vi "CTL_TestController.vi"(6 "error in (no error)":errorcluster, 7 "VISA Refnum In":refnum<visa-resource-name>, 8 "TEST State In":T6, 11 "FullConfig":T7={"Bench Params"={"Relative Root Name"="PWC-OLS", "Values"={"Step Levels"=11.0, "Resistor Tolerence"=0.01, "Sample Rate"=0.05, "Resistor"=100.0, "Wait Time"=3.0}, "Report Template path"=path "PWC-OLS/$ReportFiles/ReportTemplate_03.xlsx", "Test Type"="OLS001", "Config File Name"="8005571-05 Elevate OLS .csv", "Config 2 Use"="Default", "Skip Pre Lube"=FALSE}, "Test Params"=[[98.0, 102.0, 8.5, 8.5, 8.5, 8.5, 98.0, 102.0, 8.5, 8.5, 8.5, 8.5], [98.0, 102.0, 7.91, 8.01, 7.55, 7.65, 98.0, 102.0, 7.685, 7.785, 7.325, 7.425], [197.0, 203.0, 7.46, 7.56, 7.1, 7.2, 197.0, 203.0, 7.235, 7.335, 6.875, 6.975], [296.0, 304.0, 7.01, 7.11, 6.65, 6.75, 296.0, 304.0, 6.785, 6.885, 6.425, 6.525], [395.0, 405.0, 6.56, 6.66, 6.2, 6.3, 395.0, 405.0, 6.335, 6.435, 5.975, 6.075], [494.0, 506.0, 6.11, 6.21, 5.75, 5.85, 494.0, 506.0, 5.885, 5.985, 5.525, 5.625], [593.0, 607.0, 5.66, 5.76, 5.3, 5.4, 593.0, 607.0, 5.435, 5.535, 5.075, 5.175], [692.0, 708.0, 5.21, 5.31, 4.85, 4.95, 692.0, 708.0, 4.985, 5.085, 4.625, 4.725], [791.0, 809.0, 4.76, 4.86, 4.4, 4.5, 791.0, 809.0, 4.535, 4.635, 4.175, 4.275], [890.0, 910.0, 4.31, 4.41, 3.95, 4.05, 890.0, 910.0, 4.085, 4.185, 3.725, 3.825], [989.0, 1011.0, 3.86, 3.96, 3.5, 3.6, 989.0, 1011.0, 3.635, 3.735, 3.275, 3.375], [1088.0, 1112.0, 3.41, 3.51, 3.05, 3.15, 1088.0, 1112.0, 3.185, 3.285, 2.825, 2.925], [1088.0, 1112.0, 2.5, 2.5, 2.5, 2.5, 1088.0, 1112.0, 2.5, 2.5, 2.5, 2.5]], "Pump Params"={"Empty Inches"=8.4, "Full Inches"=2.6, "RNG_SLOW"=0.5, "RNG_CREEP"=0.007, "RNG_STOP "=0.002, "VISA resource name"="Default", "SPD_SLOW"=1, "SPD_CREEP"=0, "SPD_FAST"=5, "Zero template"=path "30", "zero  Settle sec"=100, "Laser Slope"=-0.996, "Laser Offset"=9.601, "Sim Fill Rate"=0.002, "Cal Date"="CAL_Level_RnR_241105.xlsx", "Cal Technician"="7"}, "DataQ Params"={"Visa Name"="COM4", "Num Chan"=2, "Cal Coef"=[{"M"=175.33, "B"=2.65678}, {"M"=174.448, "B"=3.00272}, {"M"=175.0, "B"=3.0}, {"M"=175.0, "B"=3.0}, {"M"=175.0, "B"=3.0}, {"M"=175.0, "B"=3.0}, {"M"=175.0, "B"=3.0}, {"M"=175.0, "B"=3.0}], "Scale "=2, "Cal Date"="1/26/2024", "Cal Technicain"="Default"}, "Pump Control Ref"={"Fill "=refnum, "Drain"=refnum, "Level PV"=refnum, "Pump Speed"=refnum, "Run Test"=refnum, "Sim"=refnum, "Jog"=refnum, "Level SP"=refnum}, "Bench Status"={"Pump Status"=refnum, "Dataq Status"=refnum, "LaserStatus"=refnum}} {"Pump Params"."Sim Fill Rate" format="%.3f"; "Pump Params"."Laser Offset" format="%.3f"; "Pump Params"."Laser Slope" format="%.3f"; "Pump Params"."RNG_STOP" format="%#_13g"; "Pump Params"."RNG_CREEP" format="%#_13g"; "Pump Params"."RNG_SLOW" format="%#_13g"}) -> (0 "TEST State Out":T6, 1 "Enable":bool, 2 "Level Out":T1={"Laser "={"Raw"=0.0, "Scaled"=0.0}, "Level PV"=9.399999618530273, "Fill"=FALSE, "Drain"=FALSE}, 3 "Specs Out":T2={"aSpecsTable"=[], "Pump CtlRef In"={"Fill "=refnum, "Drain"=refnum, "Level PV"=refnum, "Pump Speed"=refnum, "Run Test"=refnum, "Sim"=refnum, "Jog"=refnum, "Level SP"=refnum}, "TEST State Out"=enum."MANUAL", "TEST Index"=0, "Drain!Fill"=TRUE}, 4 "error out":errorcluster, 5 "Test Index Out":i32)   [LabVIEW 2024]
doc: "Simulates the level inch (0 = empty) and Level Sense (8.5 = empty).\nIf Test Status is manual then the Drain and Fill buttons cause the level to decrese or increase.\nOtherwise, drain and fill are determnied by the state variable and the difference between Level SP (Set Point) and Level PV (Present Value)\nThe level rate of change is determined by the Flow Rate setting."
uses:
  Control Definitions/Def TestState.ctl
  Control Definitions/DEF_FullConfig.ctl
  Control Definitions/DEF_BenchParams.ctl
  Control Definitions/DEF_PumpParams.ctl
  Control Definitions/DEF_DataqParams.ctl
  Control Definitions/DEF_PumpCtlRefs.ctl
  Control Definitions/Def_PumpSpeed.ctl
  Control Definitions/DEF_BenchStatus.ctl
  Control Definitions/DEF_SpecsOut.ctl
  Control Definitions/Def Spec RNG.ctl
  Control Definitions/Ded LUT_Status.ctl
  Control Definitions/DEF_LevelOut.ctl
  Control Definitions/DEF_PumpManCtl.ctl
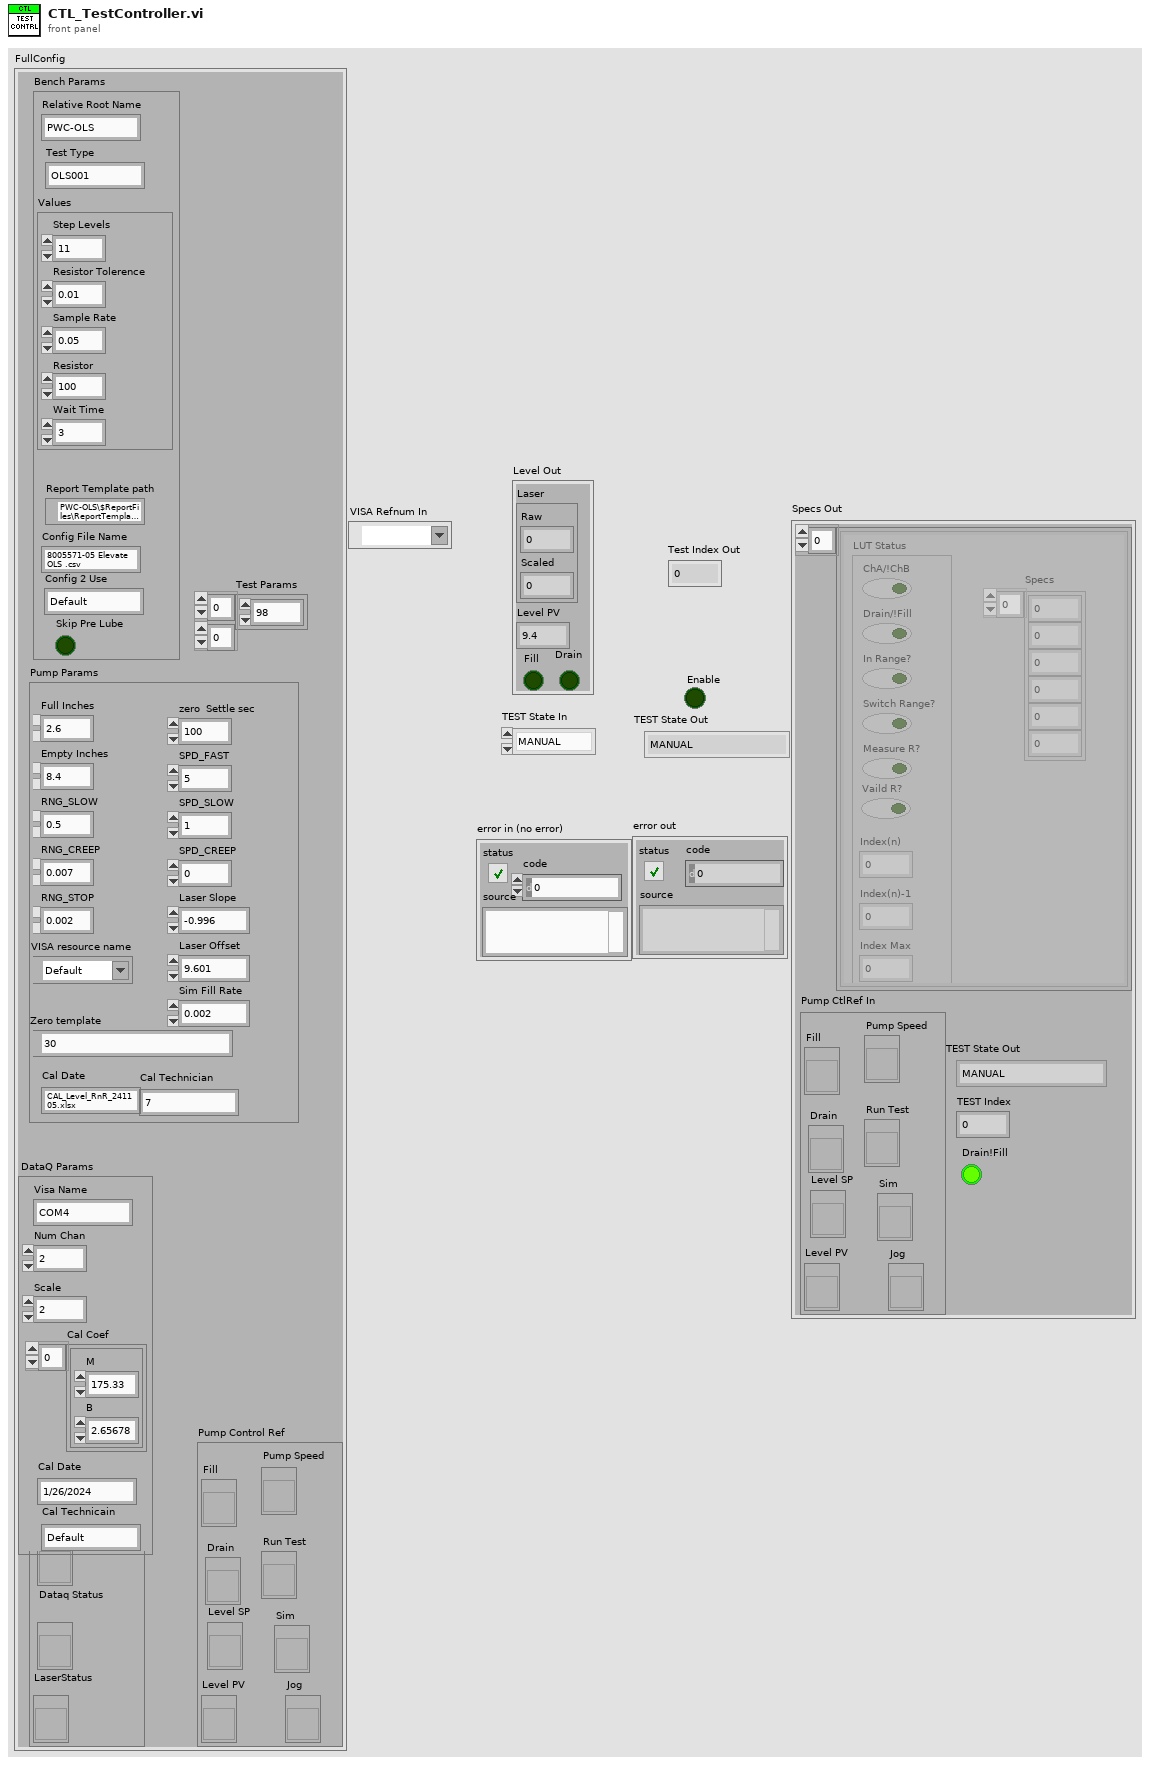
[diagram p1: front panel]
types:
  T1 = typedef "DEF_LevelOut.ctl" = cluster{"Laser ":cluster{"Raw":sgl, "Scaled":dbl}, "Level PV":dbl, "Fill":bool, "Drain":bool}
  T2 = typedef "DEF_SpecsOut.ctl" = cluster{"aSpecsTable":T3[], "Pump CtlRef In":T5, "TEST State Out":T6, "TEST Index":i32, "Drain!Fill":bool}
  T3 = typedef "Def Spec RNG.ctl" = cluster{"Specs":dbl[], "LUT Status":T4}
  T4 = typedef "Ded LUT_Status.ctl" = cluster{"ChA/!ChB":bool, "Drain/!Fill":bool, "In Range?":bool, "Switch Range?":bool, "Measure R?":bool, "Vaild R?":bool, "Index(n)":i32, "Index(n)-1":i32, "Index Max":i32, "Index(n-1)":i32}
  T5 = typedef "DEF_PumpCtlRefs.ctl" = cluster{"Fill ":refnum<vi>, "Drain":refnum<vi>, "Level PV":refnum<vi>, "Pump Speed":refnum<vi>, "Run Test":refnum<vi>, "Sim":refnum<vi>, "Jog":refnum<vi>, "Level SP":refnum<vi>}
  T6 = typedef "Def TestState.ctl" = enum16{"MANUAL", "Start", "Pre-Fill", "Pre-Fill Measure", "Pre-Drain", "Pre-Drain Measure", "Init-Record", "Load Fill Spec", "Filling Hi", "Wait1", "Record Fill", "Load Drain Spec", "Draining Lo", "Wait2", "Record Drain", "Empty", "Done"}
  T7 = typedef "DEF_FullConfig.ctl" = cluster{"Bench Params":T8, "Test Params":dbl[][], "Pump Params":T9, "DataQ Params":T10, "Pump Control Ref":T5, "Bench Status":T11}
  T8 = typedef "DEF_BenchParams.ctl" = cluster{"Relative Root Name":string, "Values":cluster{"Step Levels":dbl, "Resistor Tolerence":dbl, "Sample Rate":dbl, "Resistor":dbl, "Wait Time":dbl}, "Report Template path":path, "Test Type":string, "Config File Name":string, "Config 2 Use":string, "Skip Pre Lube":bool}
  T9 = typedef "DEF_PumpParams.ctl" = cluster{"Empty Inches":dbl, "Full Inches":dbl, "RNG_SLOW":dbl, "RNG_CREEP":dbl, "RNG_STOP ":dbl, "VISA resource name":refnum<visa-resource-name>, "SPD_SLOW":i32, "SPD_CREEP":i32, "SPD_FAST":i32, "Zero template":path, "zero  Settle sec":i32, "Laser Slope":sgl, "Laser Offset":sgl, "Sim Fill Rate":sgl, "Cal Date":string, "Cal Technician":string}
  T10 = typedef "DEF_DataqParams.ctl" = cluster{"Visa Name":string, "Num Chan":i32, "Cal Coef":cluster{"M":dbl, "B":dbl}[], "Scale ":i32, "Cal Date":string, "Cal Technicain":string}
  T11 = typedef "DEF_BenchStatus.ctl" = cluster{"Pump Status":refnum<vi>, "Dataq Status":refnum<vi>, "LaserStatus":refnum<vi>}
  T12 = typedef "DEF_PumpManCtl.ctl" = cluster{"Pump Speed":T13, "FILL":bool, "Drain":bool, "Auto/!Man":bool, "Sim Level":bool, "Raw Leve/\n!Level PVl":bool, "Jog":bool}
  T13 = typedef "Def_PumpSpeed.ctl" = enum16{"FAST", "SLOW", "CREEP", "STOP"}
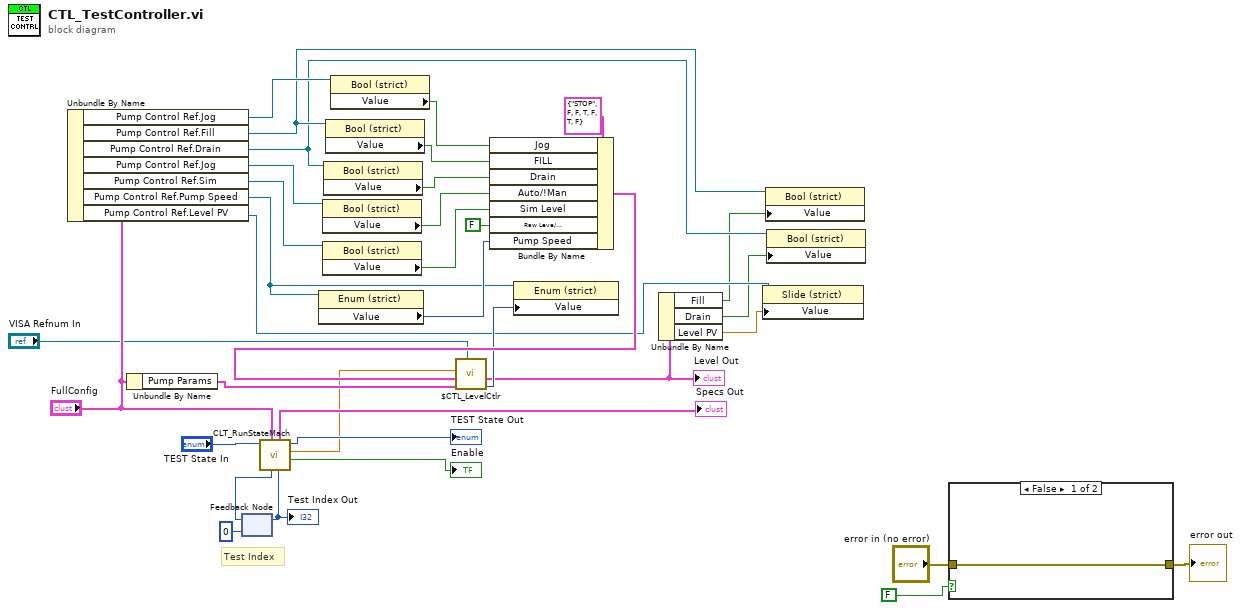
[diagram p0: block diagram]
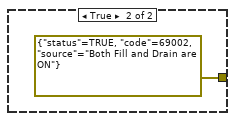
[diagram p2: hidden frame]
diagram:
  # "Test Index"
  n1 = Unbundle By Name("FullConfig") -> ("Pump Control Ref.Jog"=w7:refnum<vi>, "Pump Control Ref.Fill"=w5:refnum<vi>, "Pump Control Ref.Drain"=w4:refnum<vi>, "Pump Control Ref.Jog"=w24:refnum<vi>, "Pump Control Ref.Sim"=w23:refnum<vi>, "Pump Control Ref.Pump Speed"=w12:refnum<vi>, "Pump Control Ref.Level PV"=w10:refnum<vi>)
  n2 = Unbundle By Name("FullConfig") -> ("Pump Params"=w15:T9)
  n3 = feedback #1(0 ("Index Out")) -> (w29:i32)
  n4 = call "CLT_RunStateMach.vi"("Test Index"=w29, "FullConfig"="FullConfig", "TEST State In"="TEST State In") -> ("Enable"=→"Enable":bool, "Level S"=w14:dbl, "TEST State Out"=→"TEST State Out":T6, "Test Index Out"=w30:i32, "Specs Out"=→"Specs Out":T2)  [unwired: 4 in]
  "Test Index Out" <- w30
  n5 = feedback-in #1(w30) -> ()
  n6 = property class="Enum (strict)"(reference=w12) -> ("Value"=w13:T13)  [unwired: 1 in, 2 out]
  n7 = property class="Bool (strict)"(reference=w24) -> ("Value"=w20:bool)  [unwired: 1 in, 2 out]
  n8 = property class="Bool (strict)"(reference=w23) -> ("Value"=w19:bool)  [unwired: 1 in, 2 out]
  n9 = property class="Bool (strict)"(reference=w4) -> ("Value"=w21:bool)  [unwired: 1 in, 2 out]
  n10 = property class="Bool (strict)"(reference=w5) -> ("Value"=w22:bool)  [unwired: 1 in, 2 out]
  n11 = property class="Bool (strict)"(reference=w7) -> ("Value"=w6:bool)  [unwired: 1 in, 2 out]
  n12 = Bundle By Name(cluster=T12 {"Pump Speed"=enum."STOP", "FILL"=FALSE, "Drain"=FALSE, "Auto/!Man"=TRUE, "Sim Level"=FALSE, "Raw Leve/\n!Level PVl"=TRUE, "Jog"=FALSE} ("Pump Manual Controls"), "Jog"=w6, "FILL"=w22, "Drain"=w21, "Auto/!Man"=w20, "Sim Level"=w19, "Raw Leve/\n!Level PVl"=FALSE ("Raw Leve/\n!Level PVl"), "Pump Speed"=w13) -> (w17:T12)
  n13 = call "$CTL_LevelCtlr.vi"("VISA Refnum in"="VISA Refnum In", "Pump Params"=w15, "Pump Manual Controls"=w17, "Level SP"=w14) -> ("Pump Speed Out"=w11:T13, "Level Out"=w9:T1)  [unwired: 2 in, 4 out]
  "Level Out" <- w9
  n14 = property class="Enum (strict)"(reference=w12, "Value"=w11) -> ()  [unwired: 1 in, 2 out]
  n15 = Unbundle By Name(w9) -> ("Fill"=w2:bool, "Drain"=w3:bool, "Level PV"=w8:dbl)
  n16 = property class="Slide (strict)"(reference=w10, "Value"=w8) -> ()  [unwired: 1 in, 2 out]
  n17 = property class="Bool (strict)"(reference=w5, "Value"=w2) -> ()  [unwired: 1 in, 2 out]
  n18 = property class="Bool (strict)"(reference=w4, "Value"=w3) -> ()  [unwired: 1 in, 2 out]
  n19 = case shown="False" FALSE {
    tunnel: "error in (no error)" -> [w36 _]
    tunnel: [w36 errorcluster {"status"=TRUE, "code"=69002, "source"="Both Fill and Drain are ON"} ("error in (no error)")] -> w34
    frame False {
    }
    frame True {
    }
  }
  "error out" <- w34
